vi "1394 Color-to-Grayscale.vi"() -> ()   [LabVIEW 2011]
doc: "The Snap VI acquires an image and displays the image in an image control using low-level acquisition VIs. A snap is appropriate for low-speed or single-capture applications in which ease of programming is essential."
uses:
  <vilib>/vision/NI_Vision_Development_Module.lvlib
panel:
  in  "File Path":path
  out "Red Plane (as grayscale)":T1(plugin-control)
  out "Luminance Plane":T1(plugin-control)
  out "Original":T1(plugin-control)
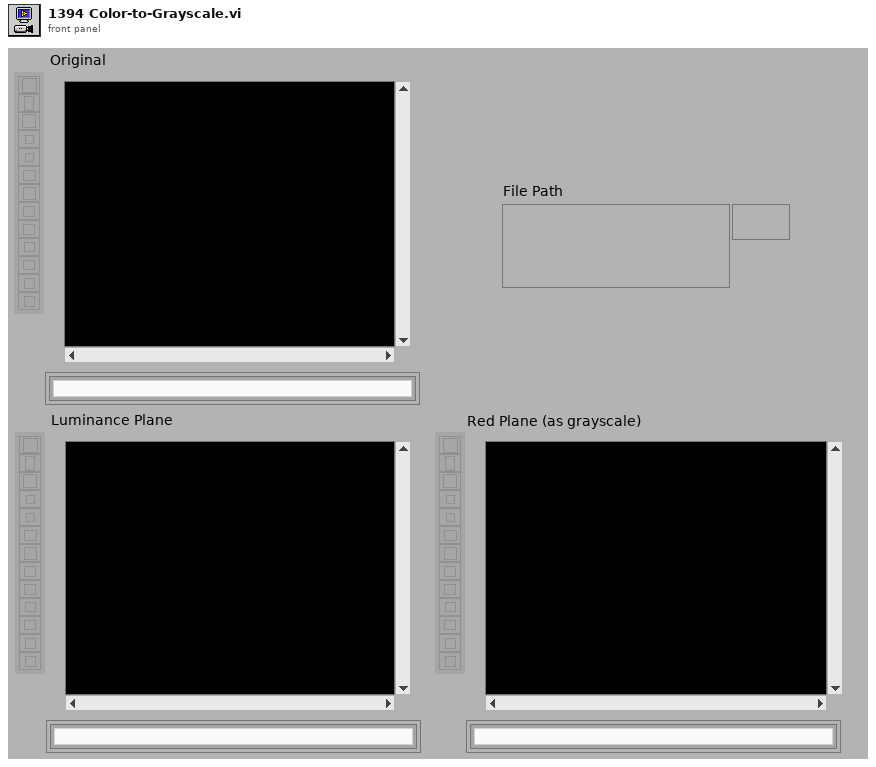
[diagram p1: front panel]
types:
  T1 = typedef "IMAQ Image.ctl" = refnum<image>
  T2 = typedef "Image Type" = u32
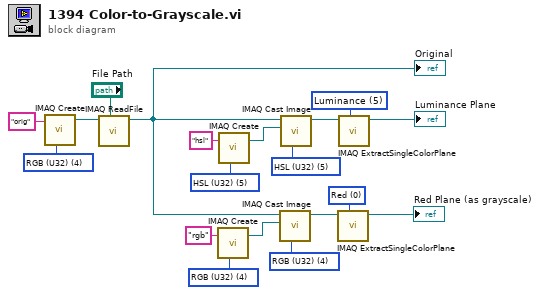
[diagram p0: block diagram]
diagram:
  w2 = T2 4 items=["Grayscale (U8)", "Grayscale (I16)", "Grayscale (SGL)", "Complex (CSG)", "RGB (U32)", "HSL (U32)", "RGB (U64)"] ("Image Type")
  w10 = 0 items=["Red", "Green", "Blue", "Hue", "Saturation", "Luminance", "Value", "Intensity"] ("Color Plane")
  w8 = T2 4 items=["Grayscale (U8)", "Grayscale (I16)", "Grayscale (SGL)", "Complex (CSG)", "RGB (U32)", "HSL (U32)", "RGB (U64)"] ("Image Type")
  w7 = T2 4 items=["Grayscale (U8)", "Grayscale (I16)", "Grayscale (SGL)", "Complex (CSG)", "RGB (U32)", "HSL (U32)", "RGB (U64)"] ("Image Type")
  w13 = 5 items=["Red", "Green", "Blue", "Hue", "Saturation", "Luminance", "Value", "Intensity"] ("Color Plane")
  w15 = T2 5 items=["Grayscale (U8)", "Grayscale (I16)", "Grayscale (SGL)", "Complex (CSG)", "RGB (U32)", "HSL (U32)", "RGB (U64)"] ("Image Type")
  w16 = T2 5 items=["Grayscale (U8)", "Grayscale (I16)", "Grayscale (SGL)", "Complex (CSG)", "RGB (U32)", "HSL (U32)", "RGB (U64)"] ("Image Type")
  n1 = call "IMAQ Create"("Image Name"="orig", "Image Type"=w2) -> ("New Image"=w4:T1)  [unwired: 3 in, 1 out]
  n2 = call "IMAQ ReadFile"("File Path"="File Path", "Image"=w4) -> ("Image Out"=w1:T1)  [unwired: 5 in, 4 out]
  "Original" <- w1
  n3 = call "IMAQ Create"("Image Name"="rgb", "Image Type"=w7) -> ("New Image"=w5:T1)  [unwired: 3 in, 1 out]
  n4 = call "IMAQ Create"("Image Name"="hsl", "Image Type"=w16) -> ("New Image"=w18:T1)  [unwired: 3 in, 1 out]
  n5 = call "IMAQ Cast Image"("Image Type"=w8, "Image Dst"=w5, "Image Src"=w1) -> ("Image Dst Out"=w9:T1)  [unwired: 7 in, 1 out]
  n6 = call "IMAQ Cast Image"("Image Type"=w15, "Image Dst"=w18, "Image Src"=w1) -> ("Image Dst Out"=w14:T1)  [unwired: 7 in, 1 out]
  n7 = call "IMAQ ExtractSingleColorPlane"("Color Plane"=w10, "Image Src"=w9) -> ("Image Dst Out"=→"Red Plane (as grayscale)":T1)  [unwired: 8 in, 1 out]
  n8 = call "IMAQ ExtractSingleColorPlane"("Color Plane"=w13, "Image Src"=w14) -> ("Image Dst Out"=→"Luminance Plane":T1)  [unwired: 8 in, 1 out]
